vi "convert thermocoupld voltage and CJC to temperature.vi"(2 "CJC R_T":sgl, 4 "ThermocoupleType":T1=6 items=["B", "E", "J", "K", "R", "S", "T", "N"], 5 "thermocouple signal":sgl) -> (0 "T_CJC":sgl, 1 "Temperature (K)":sgl format="%0.6f")   [LabVIEW 2016]
uses:
  Type Def Ctrls/RT ctrls/thermocouple type.ctl
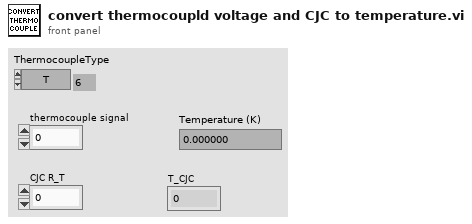
[diagram p1: front panel]
types:
  T1 = typedef "thermocouple type.ctl" = u16
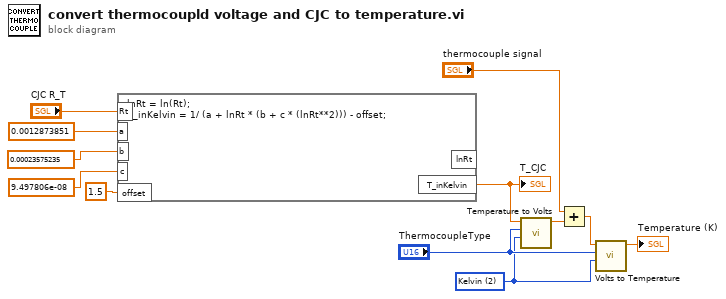
[diagram p0: block diagram]
diagram:
  w3 = u16 2 items=["Celsius", "Fahrenheit", "Kelvin", "Rankine"] ("Temperature Units")
  n1 = formula code="lnRt = ln(Rt);\nT_inKelvin = 1/ (a + lnRt * (b + c * (lnRt**2))) - offset;"("a"=0.0012873851, "b"=0.00023575235, "c"=9.497806e-08, "Rt"="CJC R_T", "offset"=1.5 ("input variable")) -> ("T_inKelvin"=w8:dbl)  [unwired: 1 out]
  "T_CJC" <- w8
  n2 = call <vilib>:"Temperature to Volts.vi"("Temperature Units"=w3, "ThermocoupleType"="ThermocoupleType", "Temperature"=w8) -> ("Thermocouple Voltage"=w7:sgl)  [unwired: 4 in]
  n3 = Add(x="thermocouple signal", y=w7) -> (x+y=w5:sgl)
  n4 = call <vilib>:"Volts to Temperature.vi"("Temperature Units"=w3, "ThermocoupleType"="ThermocoupleType", "Thermocouple Voltage"=w5) -> ("Temperature"=→"Temperature (K)":sgl)  [unwired: 4 in]
